vi "axex_sheet_exist.vi"(8 "error in":errorcluster, 10 "sheet name":string, 11 "AX Excel instance in":T1) -> (0 "error out":errorcluster, 1 "index of sheet":i32, 2 "sheet found?":bool, 3 "AX Excel instance out":T1, 4 "sheet names":string[](array[string]), 6 "sheets count":i32)   [LabVIEW 2020, in "AX Excel.lvlib"]
doc: "Call this to find out if the sheet of given name exists in current Excel file. The VI returns true if sheet is found and it also returns its index. Index -1 is returned if sheet is not found."
uses:
  AX Excel.lvlib
  axex_instance.ctl
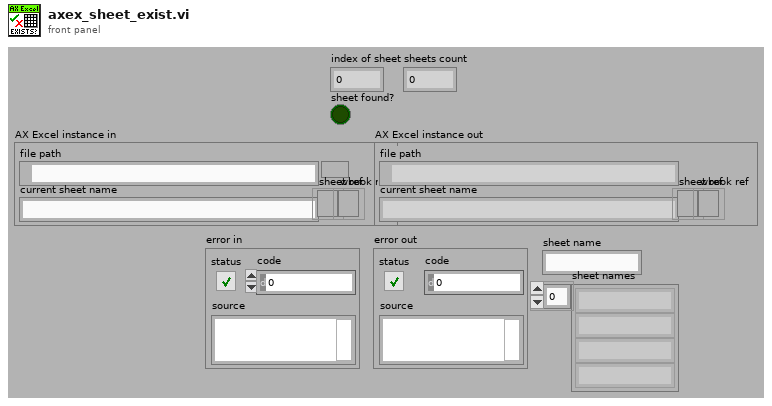
[diagram p1: front panel]
types:
  T1 = typedef "AX Excel.lvlib/axex_instance.ctl" = cluster{"file path":path, "current sheet name":string, "sheet ref":refnum<k7>, "wbook ref":refnum<k7>}
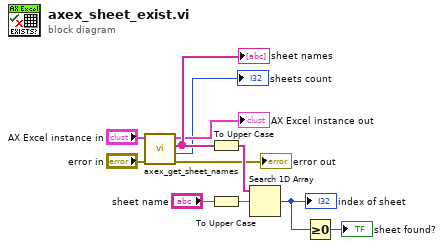
[diagram p0: block diagram]
diagram:
  n1 = call "axex_get_sheet_names.vi"("error in"="error in", "AX Excel instance in"="AX Excel instance in") -> ("error out"=→"error out":errorcluster, "sheets count"=→"sheets count":i32, "sheet names"=w9:string[], "AX Excel instance out"=→"AX Excel instance out":T1)  [unwired: 5 in, 1 out]
  "sheet names" <- w9
  n2 = To Upper Case(1:w9) -> (0:w7:string[])
  n3 = To Upper Case(1:"sheet name") -> (0:w6:string)
  n4 = Search 1D Array(1D array=w7, element=w6) -> (index of element=w5:i32)  [unwired: 1 in]
  "index of sheet" <- w5
  n5 = Greater Or Equal To 0?(x=w5) -> (x >= 0?=→"sheet found?":bool)
